vi "log_simple.vi"(4 "errorMsg":string="URL=", 7 "URL":string="URL=", 8 "StartTime":string, 11 "采集项":string[](array[string])) -> ()   [LabVIEW 2015]
uses:
  <vilib>/Utility/file.llb/Write Delimited Spreadsheet (string).vi
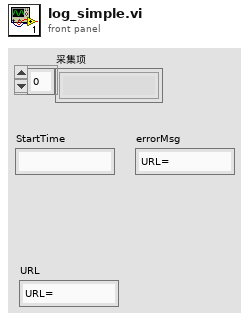
[diagram p1: front panel]
types:
  T1 = enum16{"open", "replace", "create", "open or create", "replace or create", "replace or create with confirmation"}
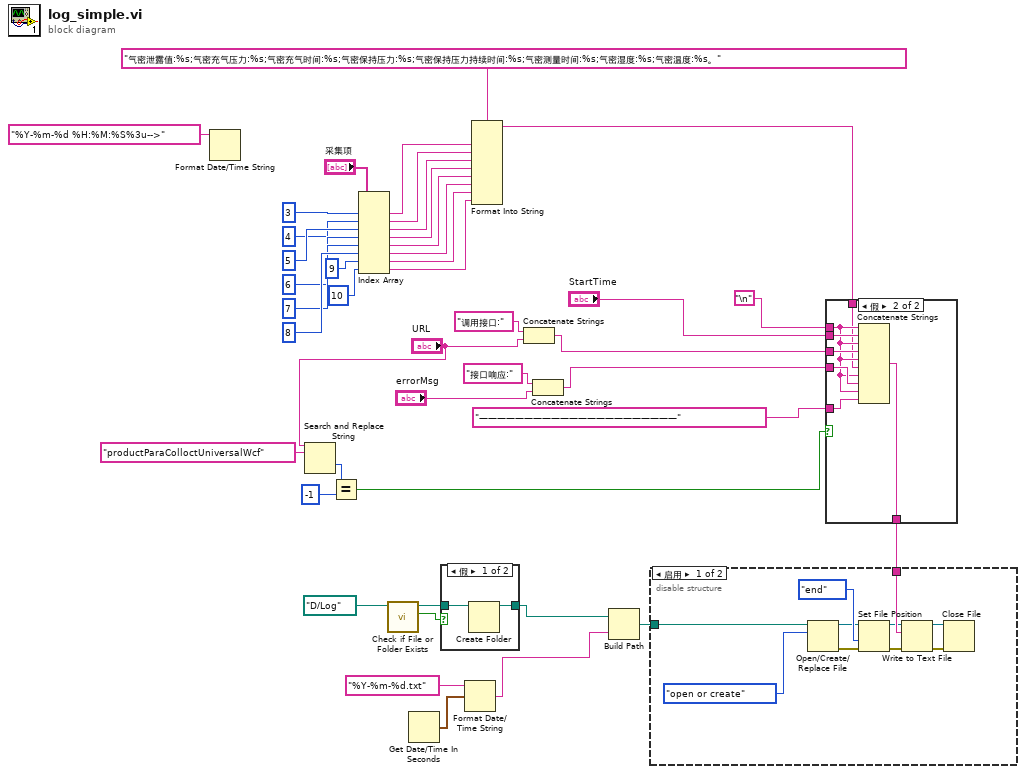
[diagram p0: block diagram]
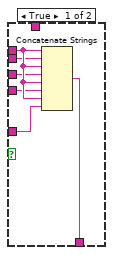
[diagram p2: hidden frame]
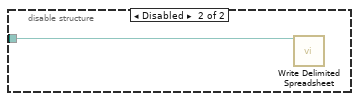
[diagram p3: hidden frame]
diagram:
  n1 = Format Date/Time String(time format string (%c)="%Y-%m-%d %H:%M:%S%3u-->" ("时间格式字符串(%c)")) -> ()  [unwired: 2 in, 1 out]
  n2 = Search and Replace String(input string="URL", search string="productParaColloctUniversalWcf" ("搜索字符串")) -> (offset past replacement=w21:i32)  [unwired: 6 in, 3 out]
  n3 = Equal?(x=w21, y=-1) -> (x = y?=w20:bool)
  n4 = Index Array(array="采集项", index #1=3 ("索引"), index #2=4 ("索引"), index #3=5 ("索引"), index #4=6 ("索引"), index #5=7 ("索引"), index #6=8 ("索引"), index #7=9 ("索引"), index #8=10 ("索引")) -> (element #1=w12:string, element #2=w11:string, element #3=w10:string, element #4=w9:string, element #5=w8:string, element #6=w7:string, element #7=w3:string, element #8=w2:string)
  n5 = call <vilib>:"Check if File or Folder Exists.vi"("path"=path "D:/Log" ("路径")) -> ("file or folder exists?"=w39:bool, "dup path"=w40:path)  [unwired: 8 in, 1 out]
  n6 = Get Date/Time In Seconds() -> (seconds since 1Jan1904=w35:timestamp)
  n7 = case shown="假" w39 {
    tunnel: w40 -> [w44 w45]
    tunnel: [w43 w45] -> w37
    frame False {
      n8 = Create Folder(path (use dialog)=w44) -> (created path=w43:path)  [unwired: 2 in, 2 out]
    }
    frame True {
    }
  }
  n9 = Format Date/Time String(time format string (%c)="%Y-%m-%d.txt" ("时间格式字符串(%c)"), seconds (now)=w35) -> (date/time string=w34:string)  [unwired: 1 in]
  n10 = Format Into String(format string="气密泄露值:%s;气密充气压力:%s;气密充气时间:%s;气密保持压力:%s;气密保持压力持续时间:%s;气密测量时间:%s;气密湿度:%s;气密温度:%s。" ("value"), w12, w11, w10, w9, w8, w7, w3, w2) -> (resulting string=w6:string)  [unwired: 2 in, 1 out]
  n11 = Concatenate Strings("调用接口:" ("value"), "URL") -> (w30:string)
  n12 = Concatenate Strings("接口响应:" ("value"), "errorMsg") -> (w27:string)
  n13 = Build Path(base path=w37, name or relative path=w34) -> (appended path=w41:path)
  n14 = case shown="假" w20 {
    tunnel: [w51 w58] -> w42
    tunnel: "\n" -> [w50 w53]
    tunnel: "StartTime" -> [w49 w57]
    tunnel: w30 -> [w48 w56]
    tunnel: w27 -> [w47 w55]
    tunnel: "——————————————————————" ("value") -> [w46 w54]
    tunnel: w6 -> [_ w52]
    frame True {
      n15 = Concatenate Strings(w50, w49, w50, w48, w50, w47, w50, w46) -> (w51:string)
    }
    frame False {
      n16 = Concatenate Strings(w53, w57, w53, w56, w53, w52, w53, w55, w53, w54) -> (w58:string)
    }
  }
  n17 = disable-structure shown="启用" {
    disable-tunnel: w42 -> [w68 _]
    disable-tunnel: w41 -> [w59 w69]
    frame Enabled {
      n18 = Open/Create/Replace File(file path (use dialog)=w59, operation (0:open)=T1."open or create" ("操作(0:open)")) -> (refnum out=w63:refnum<file>, error out=w64:errorcluster)  [unwired: 4 in, 1 out]
      n19 = Set File Position(refnum=w63, from (0:start)=enum16{"start", "end", "current"}."end" ("自（0:起始）"), error in=w64) -> (refnum out=w65:refnum<file>, error out=w66:errorcluster)  [unwired: 1 in]
      n20 = Write to Text File(file (use dialog)=w65, text=w68, error in=w66) -> (refnum out=w62:refnum<file>, error out=w61:errorcluster)  [unwired: 1 in, 1 out]
      n21 = Close File(refnum=w62, error in=w61) -> ()  [unwired: 2 out]
    }
    frame Disabled {
      n22 = call-poly <vilib>:"Write Delimited Spreadsheet.vi"("file path (dialog if empty)"=w69) -> ()  [unwired: 13 in, 2 out]
    }
  }
